vi "superKPortUtilU32.vi"(5 "WriteNotRead":bool, 6 "Register":u8, 7 "Destination":u8, 8 "error in (no error)":errorcluster, 10 "U16in":u16, 11 "VISA Refnum in":refnum<visa-resource-name>) -> (0 "error out":errorcluster, 2 "[U16]":u16[](array[numeric]), 3 "VISA Refnum out":refnum<visa-resource-name>)   [LabVIEW 2015]
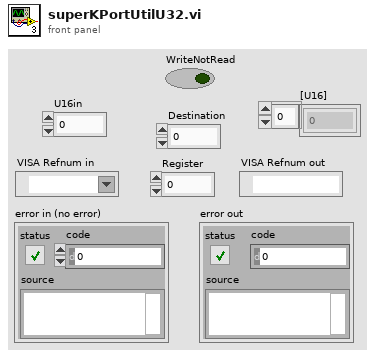
[diagram p1: front panel]
types:
  T1 = cluster{"Destination":u8, "Source":u8, "Register":u8, "Array":i16[], "WriteNotRead":bool, "ReadWithPreample":bool, "Ring":u16, "String":string, "Long":i32}
  T2 = cluster{"OpenPort":bool, "ClosePort":bool, "Baudrate":i32, "Wait":u16, "ReadWrite":bool}
  T3 = cluster{"Source":u8, "TelegramType":u8, "Register":u8, "Destination":u8, "TelegramReceived":bool, "CRC error":bool, "PayloadByteArray":u8[], "(hi.lo)":u16, "Crc16":u16, "Long":i32, "PayloadIntArray":u16[], "String":string}
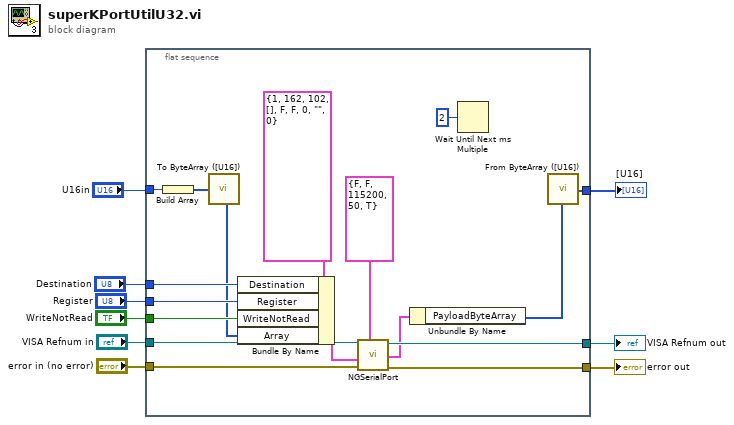
[diagram p0: block diagram]
diagram:
  n1 = flat-sequence {
    tunnel: "WriteNotRead" -> [w24]
    tunnel: "Destination" -> [w22]
    tunnel: "Register" -> [w21]
    tunnel: [w20] -> w6
    tunnel: [w19] -> w5
    tunnel: "error in (no error)" -> [w18]
    tunnel: "VISA Refnum in" -> [w17]
    tunnel: [w13] -> w2
    tunnel: "U16in" -> [w12]
    frame #0 {
      n2 = Build Array(w12) -> (w11:u16[])
      n3 = call "To ByteArray ([U16]).vi"("[U16]"=w11) -> ("PayloadByteArray"=w10:u8[])
      n4 = Bundle By Name(cluster=T1 {"Destination"=1, "Source"=162, "Register"=102, "Array"=[], "WriteNotRead"=FALSE, "ReadWithPreample"=FALSE, "Ring"=0, "String"="", "Long"=0} ("InParameters"), "Destination"=w22, "Register"=w21, "WriteNotRead"=w24, "Array"=w10) -> (w23:T1)
      n5 = call "NGSerialPort.vi"("PortParameters"=T2 {"OpenPort"=FALSE, "ClosePort"=FALSE, "Baudrate"=115200, "Wait"=50, "ReadWrite"=TRUE}, "error in"=w18, "InParameters"=w23, "VISA in"=w17) -> ("error out"=w20:errorcluster, "OutParameters"=w16:T3, "VISA out"=w19:refnum<visa-resource-name>)  [unwired: 5 in]
      n6 = Unbundle By Name(w16) -> ("PayloadByteArray"=w14:u8[])
      n7 = Wait Until Next ms Multiple(millisecond multiple=u32 2) -> ()  [unwired: 1 out]
      n8 = call "From ByteArray ([U16]).vi"("PayloadByteArray"=w14) -> ("[U16]"=w13:u16[])
    }
  }
  "error out" <- w6
  "VISA Refnum out" <- w5
  "[U16]" <- w2
